vi "test.vi"() -> ()   [LabVIEW 2023]
panel:
  out "x > y?":bool
  out "inElement":string
  out "memoString":string
  in  "Transaction Type":T1(ring)
  in  "file path":path
  out "inString":string
  out "ArrayOut":string[](array[string])
  out "Array":string[](array[string])
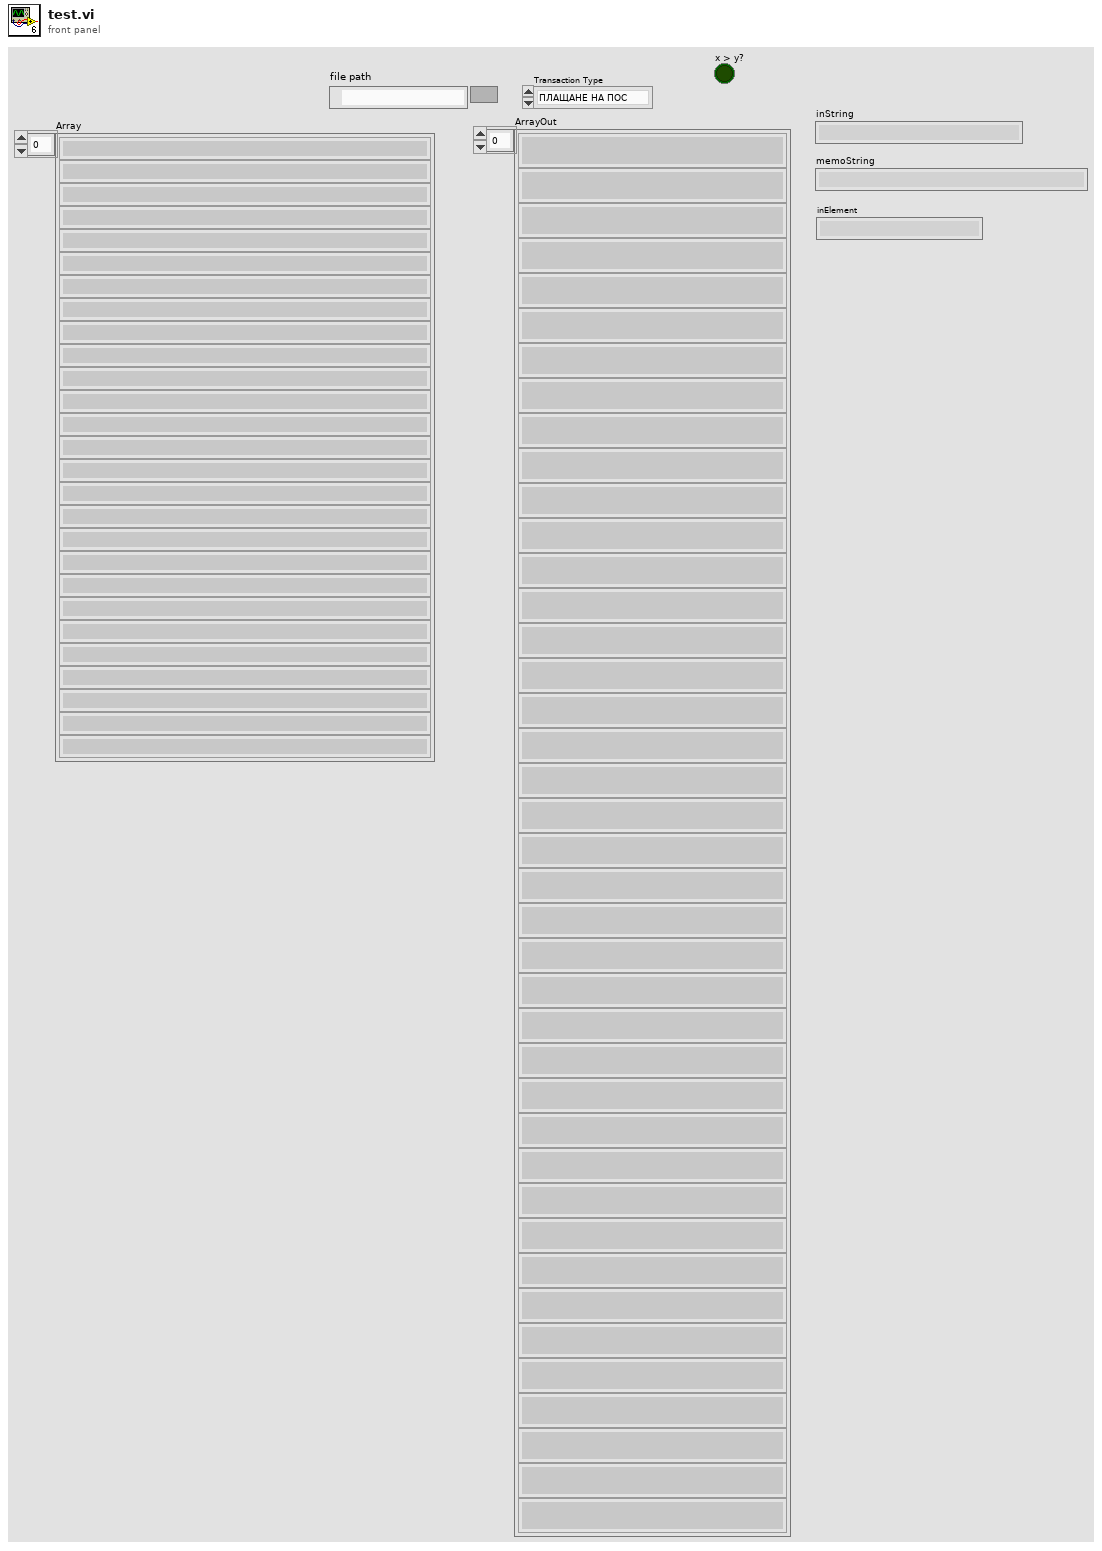
[diagram p1: front panel]
types:
  T1 = enum16{"ПЛАЩАНЕ НА ПОС", "СБКО", "ТЕГЛЕНЕ", "ЗАЕМ", "BREZOVO", "VIVACOM", "ЕЛЕКТРОХОЛД", "ЕВН", "ЗАПЛАТА", "АВАНС", "НЕТ", "ТРАНСФЕР"}
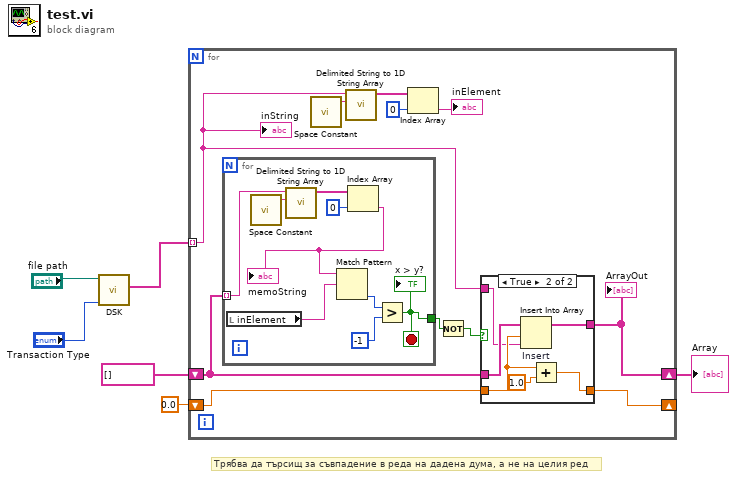
[diagram p0: block diagram]
diagram:
  # "Трябва да търсищ за съвпадение в реда на дадена дума, а не на целия ред"
  n1 = call "DSK.vi"("Transaction Type"="Transaction Type", "file path"="file path") -> ("Array 3"=w1:string[])  [unwired: 6 in, 3 out]
  n2 = for {
    shift-right: [w17] -> _
    shift-left: 0.0 ("y") -> [w16]
    tunnel: w1 -> [w10] mode=indexing
    shift-right: [w15] -> w6
    shift-left: string[] [] -> [w12]
    n3 = for {
      tunnel: w12 -> [w20] mode=indexing
      tunnel: [w23] -> w14
      stop <- w23 stop-if-true
      n4 = local read "inElement"() -> (w25:string)
      n5 = call <vilib>:"Space Constant.vi"() -> ("String"=w21:string)
      n6 = call <vilib>:"Delimited String to 1D String Array.vi"("delimiter"=w21, "delimited string"=w20) -> ("string array"=w19:string[])  [unwired: 9 in]
      n7 = Index Array(array=w19, index=0) -> (element=w18:string)
      "memoString" <- w18
      n8 = Match Pattern(string=w18, regular expression=w25) -> (offset past match=w24:i32)  [unwired: 1 in, 3 out]
      n9 = Greater?(x=w24, y=-1 ("offset past replacement")) -> (0:w23:bool)
      "x > y?" <- w23
    }
    n10 = call <vilib>:"Space Constant.vi"() -> ("String"=w11:string)
    n11 = call <vilib>:"Delimited String to 1D String Array.vi"("delimiter"=w11, "delimited string"=w10) -> ("string array"=w9:string[])  [unwired: 9 in]
    n12 = Index Array(array=w9, index=0) -> (element=→"inElement":string)
    n13 = Not(x=w14) -> (.not. x?=w13:bool)
    n14 = case shown="True" w13 {
      tunnel: [w28 w33] -> w17
      tunnel: w16 -> [w28 w32]
      tunnel: [w27 w31] -> w15
      tunnel: w12 -> [w27 w30]
      tunnel: w10 -> [_ w29]
      frame False {
      }
      frame True {
        n15 = Insert Into Array "Insert"(array=w30, index=w32, new element=w29) -> (w31:string[])
        n16 = Add(x=w32, y=1.0) -> (x+y=w33:dbl)
      }
    }
    "ArrayOut" <- w15
    "inString" <- w10
  }
  "Array" <- w6
